vi "RemoteLogCore.vi"(11 "LoggerMonitorControlData":T1) -> ()   [LabVIEW 2016]
uses:
  LoggerMonitorControlData.ctl
  General/RemoteFiles/connectionData.ctl
  General/CorePluginInfo.ctl
panel:
  out "consoleData":string
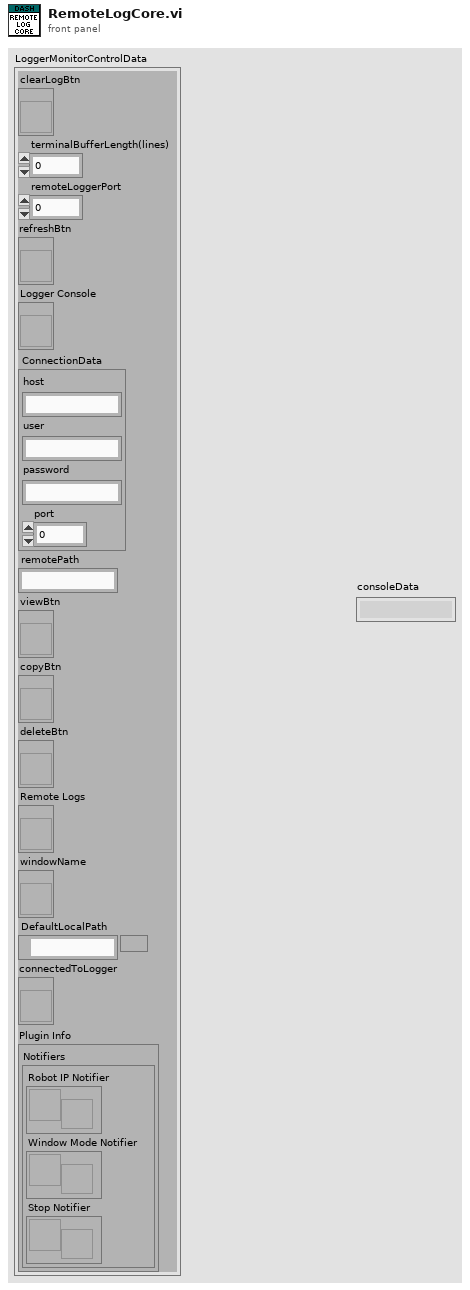
[diagram p1: front panel]
types:
  T1 = typedef "LoggerMonitorControlData.ctl" = cluster{"clearLogBtn":refnum<vi>, "terminalBufferLength(lines)":i32, "remoteLoggerPort":u16, "refreshBtn":refnum<vi>, "Logger Console":refnum<vi>, "ConnectionData":T2, "remotePath":string, "viewBtn":refnum<vi>, "copyBtn":refnum<vi>, "deleteBtn":refnum<vi>, "Remote Logs":refnum<vi>, "windowName":refnum<vi>, "DefaultLocalPath":path, "connectedToLogger":refnum<vi>, "Plugin Info":T3}
  T2 = typedef "connectionData.ctl" = cluster{"host":string, "user":string, "password":string, "port":u16}
  T3 = typedef "CorePluginInfo.ctl" = cluster{"Notifiers":cluster{"Robot IP Notifier":refnum<notifier>, "Window Mode Notifier":refnum<notifier>, "Stop Notifier":refnum<notifier>}}
  T4 = enum16{"Standard", "Buffered", "CRLF", "Immediate"}
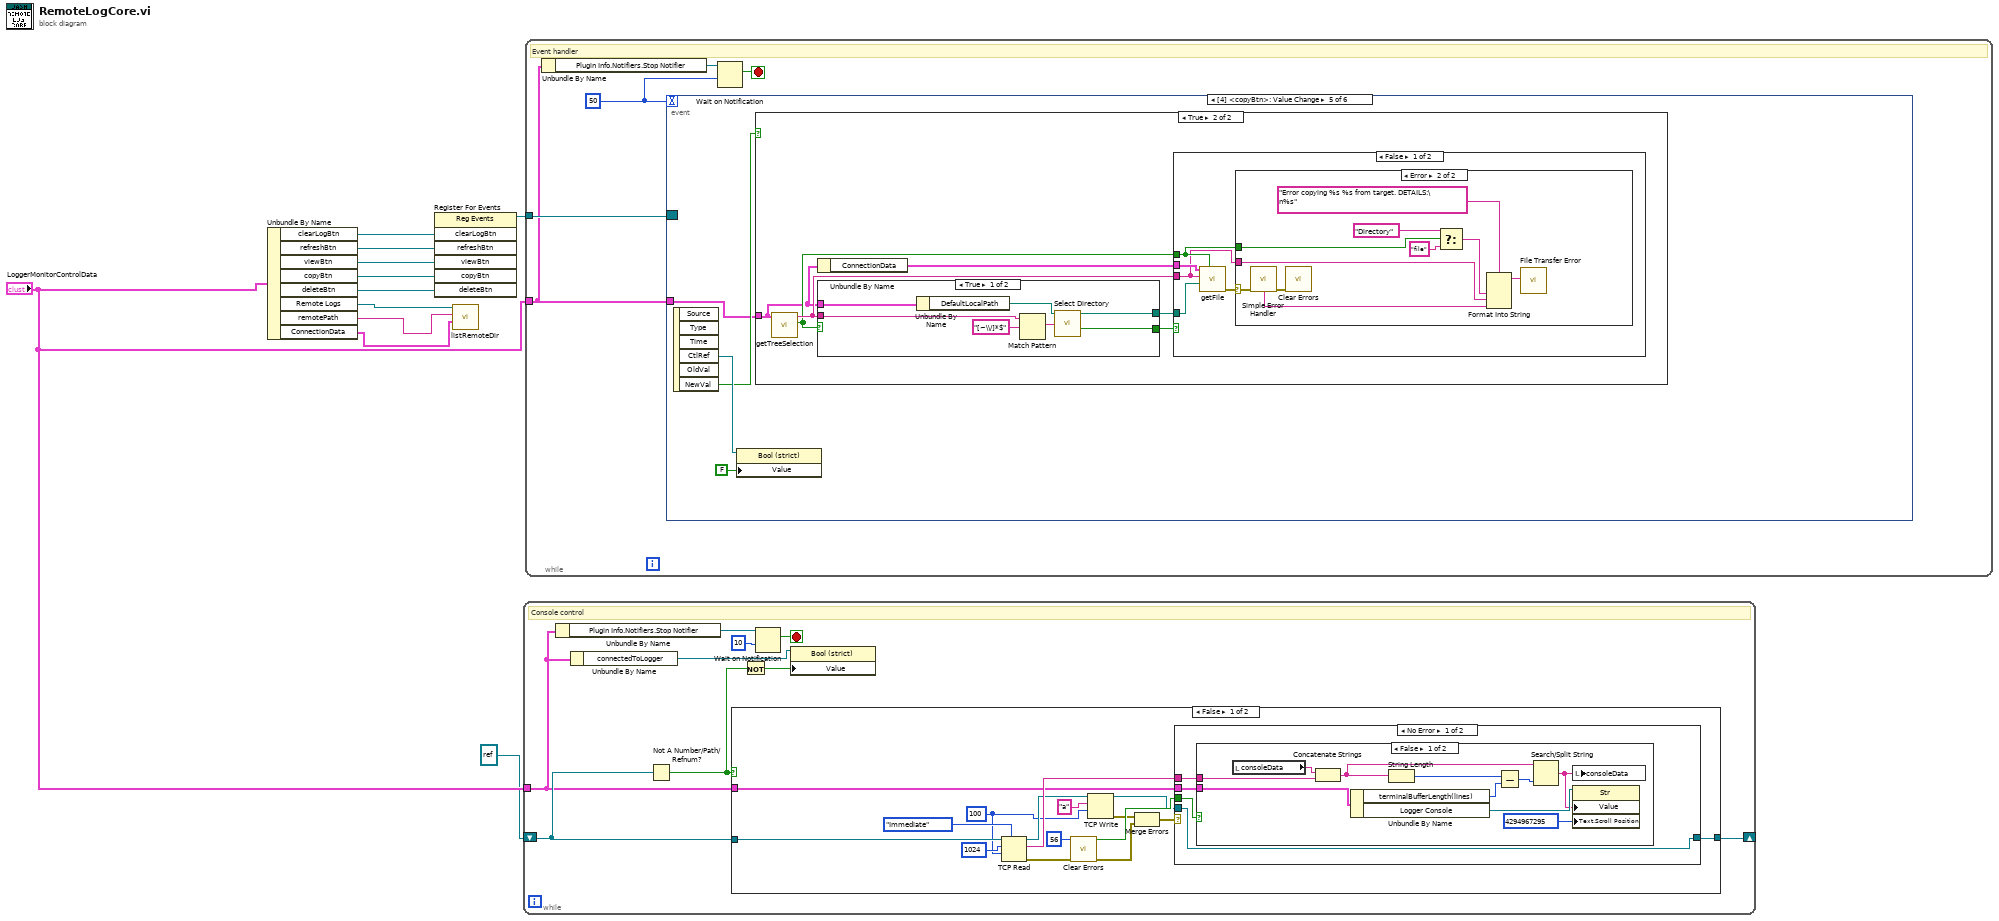
[diagram p0: block diagram]
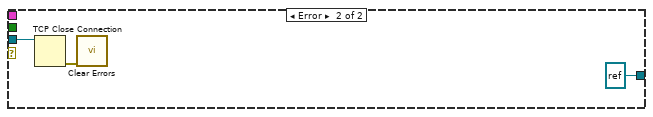
[diagram p3: hidden frame]
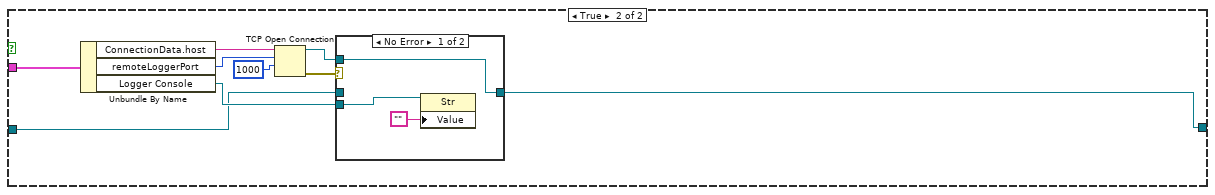
[diagram p4: hidden frame]
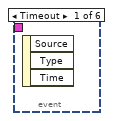
[diagram p6: hidden frame]
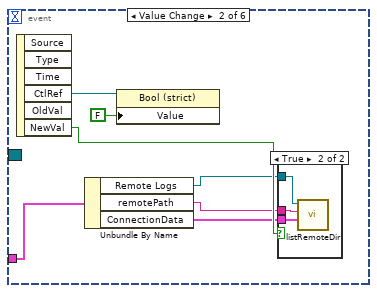
[diagram p7: hidden frame]
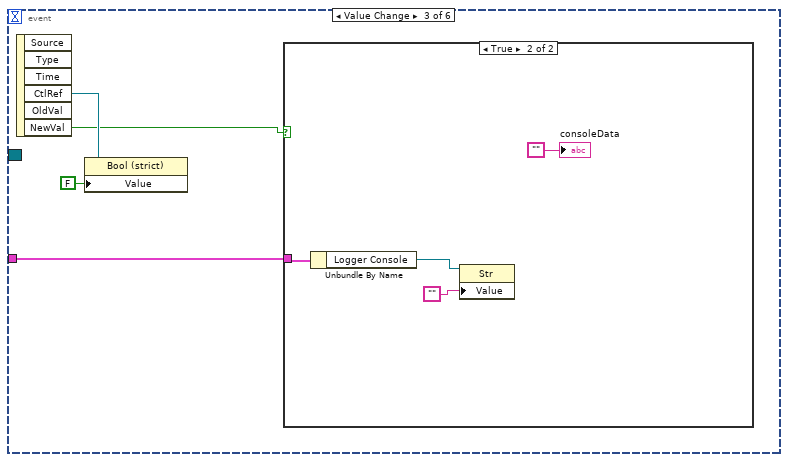
[diagram p9: hidden frame]
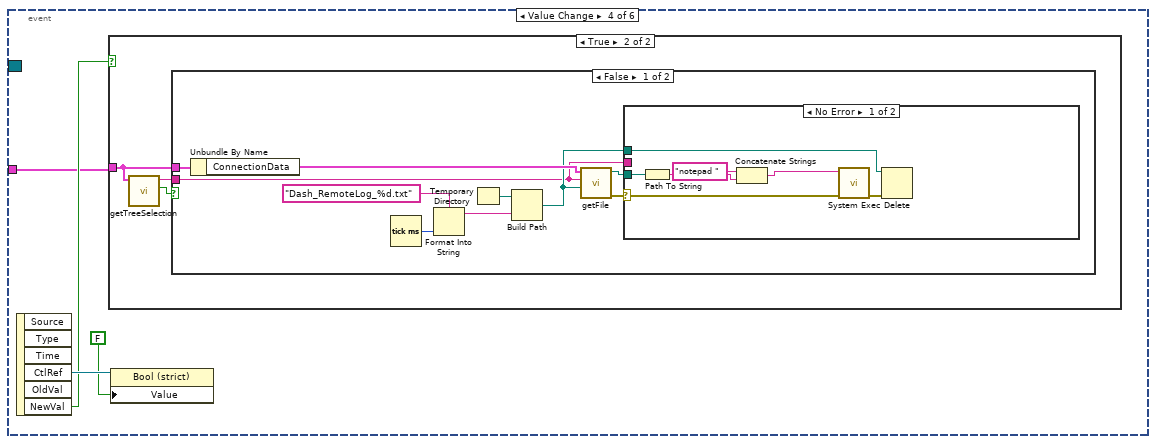
[diagram p11: hidden frame]
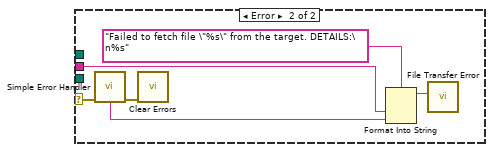
[diagram p13: hidden frame]
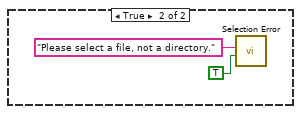
[diagram p14: hidden frame]
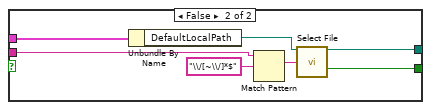
[diagram p16: hidden frame]
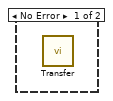
[diagram p17: hidden frame]
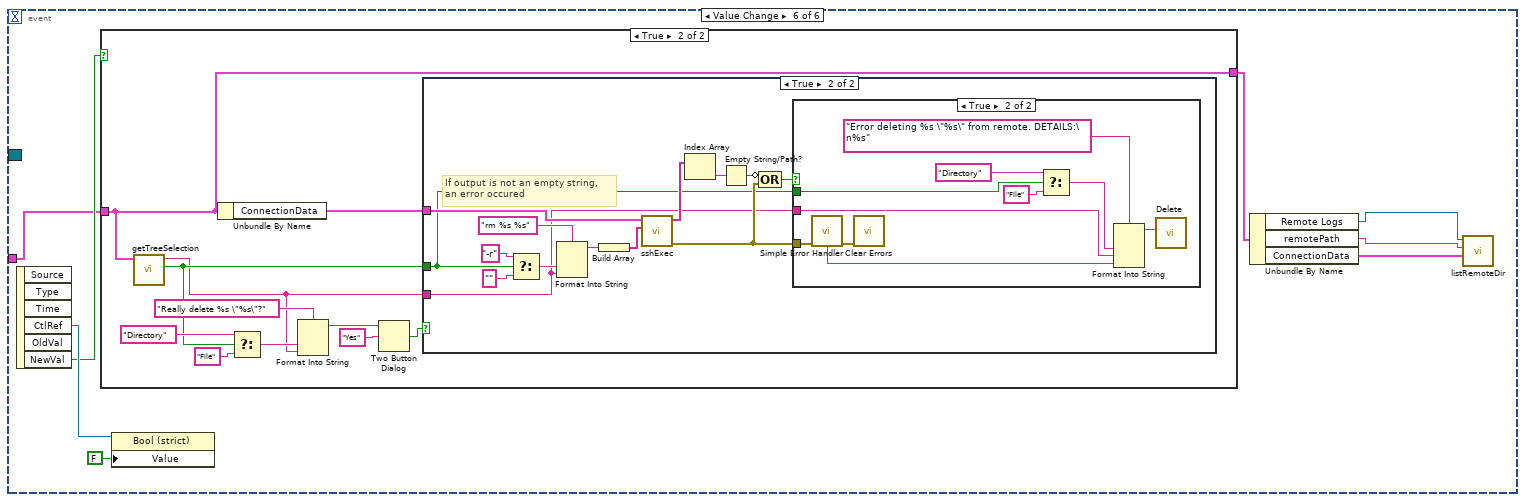
[diagram p19: hidden frame]
diagram:
  n1 = Unbundle By Name("LoggerMonitorControlData") -> ("clearLogBtn"=w11:refnum<vi>, "refreshBtn"=w10:refnum<vi>, "viewBtn"=w9:refnum<vi>, "copyBtn"=w8:refnum<vi>, "deleteBtn"=w7:refnum<vi>, "Remote Logs"=w3:refnum<vi>, "remotePath"=w1:string, "ConnectionData"=w2:T2)
  n2 = register-events(w11, w10, w9, w8, w7) -> (reference out=w6:refnum<event-registration>)  [unwired: 2 in, 1 out]
  n3 = call "listRemoteDir.vi"("ConnectionData"=w2, "remote path"=w1, "TreeControlRefIn"=w3) -> ()  [unwired: 7 in, 2 out]
  n4 = while {
    tunnel: "LoggerMonitorControlData" -> [w15]
    shift-right: [w17] -> _
    shift-left: refnum<k5> refnum ("TCPConnection") -> [w16]
    stop <- w12 stop-if-true
    # "Console control"
    n5 = Unbundle By Name(w15) -> ("Plugin Info.Notifiers.Stop Notifier"=w14:refnum<notifier>)
    n6 = Unbundle By Name(w15) -> ("connectedToLogger"=w20:refnum<vi>)
    n7 = Not A Number/Path/Refnum?(number/path/refnum=w16) -> (NaN/Path/Refnum?=w18:bool)
    n8 = case shown="False" w18 {
      tunnel: w15 -> [w30 w62]
      tunnel: [w33 w55] -> w17
      tunnel: w16 -> [w36 w54]
      frame False {
        w24 = 100 ("timeout ms (25000)")
        n9 = TCP Read(connection ID=w36, bytes to read=1024, 7:T4."Immediate" ("mode (standard)"), 9:w24) -> (connection ID out=w27:refnum<k5>, data out=w31:string, error out=w35:errorcluster)  [unwired: 1 in]
        n10 = call <vilib>:"Clear Errors.vi"("error in (no error)"=w35, "specific error code to clear (0: all)"=56) -> ("error out"=w23:errorcluster, "specific error cleared?"=w32:bool)  [unwired: 4 in]
        n11 = TCP Write(connection ID=w27, data in="a", 9:w24) -> (connection ID out=w26:refnum<k5>, error out=w22:errorcluster)  [unwired: 1 in, 1 out]
        n12 = Merge Errors(w22, w23) -> (w21:errorcluster)
        n13 = case shown="No Error" w21 {
          tunnel: [w37 refnum<k5> refnum ("TCPConnection")] -> w33
          tunnel: w32 -> [w40 _]
          tunnel: w31 -> [w39 _]
          tunnel: w30 -> [w38 _]
          tunnel: w26 -> [w37 w51]
          frame No Error {
            n14 = case shown="False" w40 {
              tunnel: w39 -> [w41 _]
              tunnel: w38 -> [w50 _]
              frame False {
                n15 = local read "consoleData"() -> (w47:string)
                n16 = Concatenate Strings(w47, w41) -> (w46:string)
                n17 = Unbundle By Name(w50) -> ("terminalBufferLength(lines)"=w42:i32, "Logger Console"=w49:refnum<vi>)
                n18 = String Length(string=w46) -> (length=w43:i32)
                n19 = Subtract(x=w43, y=w42) -> (x-y=w45:i32)
                n20 = Search/Split String(string=w46, offset (0)=w45) -> (match + rest of string=w44:string)  [unwired: 1 in, 2 out]
                n21 = local write "consoleData"(w44) -> ()
                n22 = property class="Str"(reference=w49, "Value"=w44, "Text.Scroll Position"=u32 4294967295) -> ()  [unwired: 1 in, 2 out]
              }
              frame True {
                # "If true, a timeout occured. Just keep going"
              }
            }
          }
          frame Error {
            n23 = TCP Close Connection(connection ID=w51) -> (error out=w53:errorcluster)  [unwired: 2 in, 1 out]
            n24 = call <vilib>:"Clear Errors.vi"("error in (no error)"=w53) -> ()  [unwired: 5 in, 2 out]
          }
        }
      }
      frame True {
        n25 = Unbundle By Name(w62) -> ("ConnectionData.host"=w61:string, "remoteLoggerPort"=w60:u16, "Logger Console"=w56:refnum<vi>)
        n26 = TCP Open Connection(address=w61, remote port or service name=w60, timeout ms (60000)=1000) -> (connection ID=w57:refnum<k5>, error out=w58:errorcluster)  [unwired: 2 in]
        n27 = case shown="No Error" w58 {
          tunnel: w57 -> [w63 _]
          tunnel: w56 -> [w65 _]
          tunnel: [w63 w66] -> w55
          tunnel: w54 -> [_ w66]
          frame No Error {
            n28 = property class="Str"(reference=w65, "Value"="") -> ()  [unwired: 1 in, 2 out]
          }
          frame Error {
          }
        }
      }
    }
    n29 = Not(x=w18) -> (.not. x?=w19:bool)
    n30 = Wait on Notification(notifier=w14, timeout in ms (-1)=10) -> (notification=w12:bool)  [unwired: 2 in, 3 out]
    n31 = property class="Bool (strict)"(reference=w20, "Value"=w19) -> ()  [unwired: 1 in, 2 out]
  }
  n32 = while {
    tunnel: w6 -> [w71]
    tunnel: "LoggerMonitorControlData" -> [w69]
    stop <- w70 stop-if-true
    w67 = 50
    # "Event handler"
    n33 = Unbundle By Name(w69) -> ("Plugin Info.Notifiers.Stop Notifier"=w68:refnum<notifier>)
    n34 = event shown="[4] <copyBtn>: Value Change" {
      selector: w71 -> [_ _ _ _ _ _]
      dyn-events: _ -> [_ _ _ _ _ _]
      timeout: w67 -> [_ _ _ _ _ _]
      tunnel: w69 -> [_ w77 w82 w90 w122 w165]
      event Timeout {
        n35 = event-data() -> ()  [unwired: 1 in, 3 out]
      }
      event Value Change {
        n36 = event-data() -> ("CtlRef"=w74:refnum<vi>, "NewVal"=w78:bool)  [unwired: 1 in, 4 out]
        n37 = Unbundle By Name(w77) -> ("Remote Logs"=w76:refnum<vi>, "remotePath"=w72:string, "ConnectionData"=w75:T2)
        n38 = property class="Bool (strict)"(reference=w74, "Value"=FALSE) -> ()  [unwired: 1 in, 2 out]
        n39 = case shown="True" w78 {
          tunnel: w76 -> [_ w81]
          tunnel: w75 -> [_ w80]
          tunnel: w72 -> [_ w79]
          frame False {
          }
          frame True {
            n40 = call "listRemoteDir.vi"("ConnectionData"=w80, "remote path"=w79, "TreeControlRefIn"=w81) -> ()  [unwired: 7 in, 2 out]
          }
        }
      }
      event Value Change {
        n41 = event-data() -> ("CtlRef"=w85:refnum<vi>, "NewVal"=w83:bool)  [unwired: 1 in, 4 out]
        n42 = property class="Bool (strict)"(reference=w85, "Value"=FALSE) -> ()  [unwired: 1 in, 2 out]
        n43 = case shown="True" w83 {
          tunnel: w82 -> [_ w89]
          frame False {
          }
          frame True {
            n44 = Unbundle By Name(w89) -> ("Logger Console"=w88:refnum<vi>)
            n45 = property class="Str"(reference=w88, "Value"="") -> ()  [unwired: 1 in, 2 out]
            "consoleData" <- ""
          }
        }
      }
      event Value Change {
        n46 = event-data() -> ("CtlRef"=w93:refnum<vi>, "NewVal"=w91:bool)  [unwired: 1 in, 4 out]
        n47 = case shown="True" w91 {
          tunnel: w90 -> [_ w94]
          frame False {
          }
          frame True {
            n48 = call "getTreeSelection.vi"("LoggerMonitorControlData"=w94) -> ("isDir?"=w96:bool, "SelectedPath"=w95:string)  [unwired: 8 in, 1 out]
            n49 = case shown="False" w96 {
              tunnel: w95 -> [w97 _]
              tunnel: w94 -> [w106 _]
              frame False {
                n50 = Unbundle By Name(w106) -> ("ConnectionData"=w105:T2)
                n51 = Tick Count (ms)() -> (millisecond timer value=w101:u32)
                n52 = Format Into String(format string="Dash_RemoteLog_%d.txt", w101) -> (resulting string=w102:string)  [unwired: 2 in, 1 out]
                n53 = Temporary Directory() -> (w104:path)
                n54 = Build Path(base path=w104, name or relative path=w102) -> (appended path=w99:path)
                n55 = call "getFile.vi"("local path"=w99, "remote path"=w97, "ConnectionData"=w105) -> ("error out"=w98:errorcluster, "local path out"=w100:path)  [unwired: 7 in]
                n56 = case shown="No Error" w98 {
                  selector: w98 -> [w110 w115]
                  tunnel: w100 -> [w113 _]
                  tunnel: w99 -> [w111 _]
                  tunnel: w97 -> [_ w117]
                  frame No Error {
                    n57 = Path To String(path=w113) -> (string=w109:string)
                    n58 = Concatenate Strings("notepad " ("string"), w109) -> (w107:string)
                    n59 = call <vilib>:"System Exec.vi"("error in (no error)"=w110, "command line"=w107) -> ("error out"=w112:errorcluster)  [unwired: 6 in, 3 out]
                    n60 = Delete(path (use dialog)=w111, error in=w112) -> ()  [unwired: 3 in, 3 out]
                  }
                  frame Error {
                    n61 = call <vilib>:"Simple Error Handler.vi"("error in (no error)"=w115) -> ("error out"=w114:errorcluster, "message"=w116:string)  [unwired: 4 in, 3 out]
                    n62 = call <vilib>:"Clear Errors.vi"("error in (no error)"=w114) -> ()  [unwired: 5 in, 2 out]
                    n63 = Format Into String(format string="Failed to fetch file \"%s\" from the target. DETAILS:\n%s", w117, w116) -> (resulting string=w118:string)  [unwired: 2 in, 1 out]
                    n64 = call "File Transfer Error"("Message"=w118) -> ()  [unwired: 9 in, 2 out]
                  }
                }
              }
              frame True {
                n65 = call "Selection Error"("Enable"=TRUE, "Message"="Please select a file, not a directory.") -> ()  [unwired: 8 in, 2 out]
              }
            }
          }
        }
        n66 = property class="Bool (strict)"(reference=w93, "Value"=FALSE) -> ()  [unwired: 1 in, 2 out]
      }
      event Value Change {
        n67 = event-data() -> ("CtlRef"=w124:refnum<vi>, "NewVal"=w123:bool)  [unwired: 1 in, 4 out]
        n68 = property class="Bool (strict)"(reference=w124, "Value"=FALSE) -> ()  [unwired: 1 in, 2 out]
        n69 = case shown="True" w123 {
          tunnel: w122 -> [_ w129]
          frame False {
          }
          frame True {
            n70 = call "getTreeSelection.vi"("LoggerMonitorControlData"=w129) -> ("isDir?"=w130:bool, "SelectedPath"=w131:string)  [unwired: 8 in, 1 out]
            n71 = Unbundle By Name(w129) -> ("ConnectionData"=w126:T2)
            n72 = case shown="True" w130 {
              tunnel: w131 -> [w137 w144]
              tunnel: w129 -> [w135 w142]
              tunnel: [w133 w140] -> w128
              tunnel: [w132 w139] -> w127
              frame True {
                n73 = Unbundle By Name(w135) -> ("DefaultLocalPath"=w134:path)
                n74 = Match Pattern(string=w137, regular expression="[~\\/]*$") -> (match substring=w136:string)  [unwired: 1 in, 3 out]
                n75 = call "Select Directory"("start path"=w134, "default name"=w136) -> ("selected path"=w132:path, "cancelled"=w133:bool)  [unwired: 10 in, 2 out]
              }
              frame False {
                n76 = Unbundle By Name(w142) -> ("DefaultLocalPath"=w141:path)
                n77 = Match Pattern(string=w144, regular expression="\\/[~\\/]*$") -> (match substring=w143:string)  [unwired: 1 in, 3 out]
                n78 = call "Select File"("start path"=w141, "default name"=w143) -> ("selected path"=w139:path, "cancelled"=w140:bool)  [unwired: 10 in, 2 out]
              }
            }
            n79 = case shown="False" w128 {
              tunnel: w130 -> [w147 _]
              tunnel: w127 -> [w149 _]
              tunnel: w131 -> [w146 _]
              tunnel: w126 -> [w150 _]
              frame False {
                n80 = call "getFile.vi"("isDir?"=w147, "local path"=w149, "remote path"=w146, "ConnectionData"=w150) -> ("error out"=w148:errorcluster)  [unwired: 6 in, 1 out]
                n81 = case shown="Error" w148 {
                  selector: w148 -> [_ w151]
                  tunnel: w147 -> [_ w153]
                  tunnel: w146 -> [_ w152]
                  frame No Error {
                    n82 = call "Transfer"() -> ()  [unwired: 10 in, 2 out]
                  }
                  frame Error {
                    n83 = call <vilib>:"Simple Error Handler.vi"("error in (no error)"=w151) -> ("error out"=w154:errorcluster, "message"=w155:string)  [unwired: 4 in, 3 out]
                    n84 = call <vilib>:"Clear Errors.vi"("error in (no error)"=w154) -> ()  [unwired: 5 in, 2 out]
                    n85 = Select(t="Directory" ("SelectedPath"), s=w153, f="file") -> (s? t:f=w157:string)
                    n86 = Format Into String(format string="Error copying %s %s from target. DETAILS:\n%s", w157, w152, w155) -> (resulting string=w156:string)  [unwired: 2 in, 1 out]
                    n87 = call "File Transfer Error"("Message"=w156) -> ()  [unwired: 9 in, 2 out]
                  }
                }
              }
              frame True {
              }
            }
          }
        }
      }
      event Value Change {
        n88 = event-data() -> ("CtlRef"=w168:refnum<vi>, "NewVal"=w166:bool)  [unwired: 1 in, 4 out]
        n89 = case shown="True" w166 {
          tunnel: w165 -> [w169 w170]
          tunnel: [w169 w170] -> w162
          frame False {
          }
          frame True {
            n90 = call "getTreeSelection.vi"("LoggerMonitorControlData"=w170) -> ("isDir?"=w172:bool, "SelectedPath"=w171:string)  [unwired: 8 in, 1 out]
            n91 = Unbundle By Name(w170) -> ("ConnectionData"=w173:T2)
            n92 = Select(t="Directory", s=w172, f="File") -> (s? t:f=w177:string)
            n93 = Format Into String(format string="Really delete %s \"%s\"?", w177, w171) -> (resulting string=w176:string)  [unwired: 2 in, 1 out]
            n94 = Two Button Dialog(message=w176, 2:"Yes" ("T button name (\"OK\")")) -> (T button?=w174:bool)  [unwired: 1 in]
            n95 = case shown="True" w174 {
              tunnel: w173 -> [_ w188]
              tunnel: w172 -> [_ w182]
              tunnel: w171 -> [_ w181]
              frame False {
              }
              frame True {
                # "If output is not an empty string, \nan error occured"
                n96 = Select(t="-r", s=w182, f="") -> (s? t:f=w191:string)
                n97 = Format Into String(format string="rm %s %s", w191, w181) -> (resulting string=w190:string)  [unwired: 2 in, 1 out]
                n98 = Build Array(w190) -> (w189:string[])
                n99 = call "sshExec.vi"("Commands"=w189, "ConnectionData"=w188) -> ("error out"=w183:errorcluster, "Output"=w187:string[])  [unwired: 8 in]
                n100 = Index Array(array=w187) -> (element=w186:string)  [unwired: 1 in]
                n101 = Empty String/Path?(string/path=w186) -> (empty?=w185:bool)
                n102 = Compound Arithmetic op=OR(invert w185, w183) -> (w184:bool)
                n103 = case shown="True" w184 {
                  tunnel: w183 -> [_ w198]
                  tunnel: w182 -> [_ w201]
                  tunnel: w181 -> [_ w199]
                  frame False {
                    n104 = call "Delete"() -> ()  [unwired: 10 in, 2 out]
                  }
                  frame True {
                    n105 = call <vilib>:"Simple Error Handler.vi"("error in (no error)"=w198) -> ("error out"=w196:errorcluster, "message"=w197:string)  [unwired: 4 in, 3 out]
                    n106 = call <vilib>:"Clear Errors.vi"("error in (no error)"=w196) -> ()  [unwired: 5 in, 2 out]
                    n107 = Select(t="Directory", s=w201, f="File") -> (s? t:f=w200:string)
                    n108 = Format Into String(format string="Error deleting %s \"%s\" from remote. DETAILS:\n%s", w200, w199, w197) -> (resulting string=w195:string)  [unwired: 2 in, 1 out]
                    n109 = call "Delete"("Message"=w195) -> ()  [unwired: 9 in, 2 out]
                  }
                }
              }
            }
          }
        }
        n110 = property class="Bool (strict)"(reference=w168, "Value"=FALSE) -> ()  [unwired: 1 in, 2 out]
        n111 = Unbundle By Name(w162) -> ("Remote Logs"=w164:refnum<vi>, "remotePath"=w161:string, "ConnectionData"=w163:T2)
        n112 = call "listRemoteDir.vi"("ConnectionData"=w163, "remote path"=w161, "TreeControlRefIn"=w164) -> ()  [unwired: 7 in, 2 out]
      }
    }
    n113 = Wait on Notification(notifier=w68, timeout in ms (-1)=w67) -> (notification=w70:bool)  [unwired: 2 in, 3 out]
  }
